vi "FlatToRichcif_plugincore_TimingOverrides.vi"(5 "OutputClusterType":T1, 11 "InputCluster":T2) -> (3 "OutputCluster":T1)   [LabVIEW 2021, in "CIF_Manager_client.lvlib"]
uses:
  cif_plugincore_TimingOverrides_Flat.ctl
  cif_plugincore_TimingOverrides.ctl
  CIF_Manager_client.lvlib
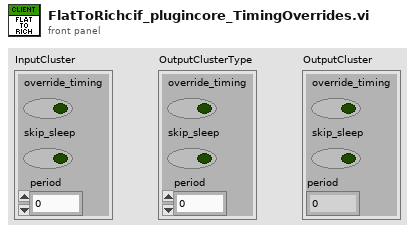
[diagram p1: front panel]
types:
  T1 = typedef "CIF_Manager_client.lvlib/cif_plugincore_TimingOverrides.ctl" = cluster{"override_timing":bool, "skip_sleep":bool, "period":dbl}
  T2 = typedef "CIF_Manager_client.lvlib/cif_plugincore_TimingOverrides_Flat.ctl" = cluster{"override_timing":bool, "skip_sleep":bool, "period":dbl}
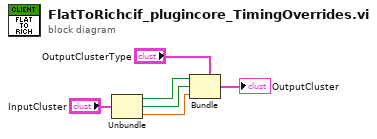
[diagram p0: block diagram]
diagram:
  n1 = Unbundle "Unbundle"("InputCluster") -> ("override_timing"=w3:bool, "skip_sleep"=w2:bool, "period"=w1:dbl)
  n2 = Bundle "Bundle"(cluster="OutputClusterType", "override_timing"=w3, "skip_sleep"=w2, "period"=w1) -> (→"OutputCluster":T1)
